vi "ModelCode_Rf.vi"(9 "BarCode":string, 11 "Data In":T1) -> (1 "ModeCode":string, 3 "Data Out":T1)   [LabVIEW 2014]
uses:
  controls/Data.ctl
panel:
  # "日期"
  # "機種名稱"
  # "機種代號"
  # "商品條碼"
  # "台"
  # "OK"
  # "NG"
  # "台"
  # "總計"
  # "台"
  # "日期"
  # "機種名稱"
  # "機種代號"
  # "商品條碼"
  # "台"
  # "OK"
  # "NG"
  # "台"
  # "總計"
  # "台"
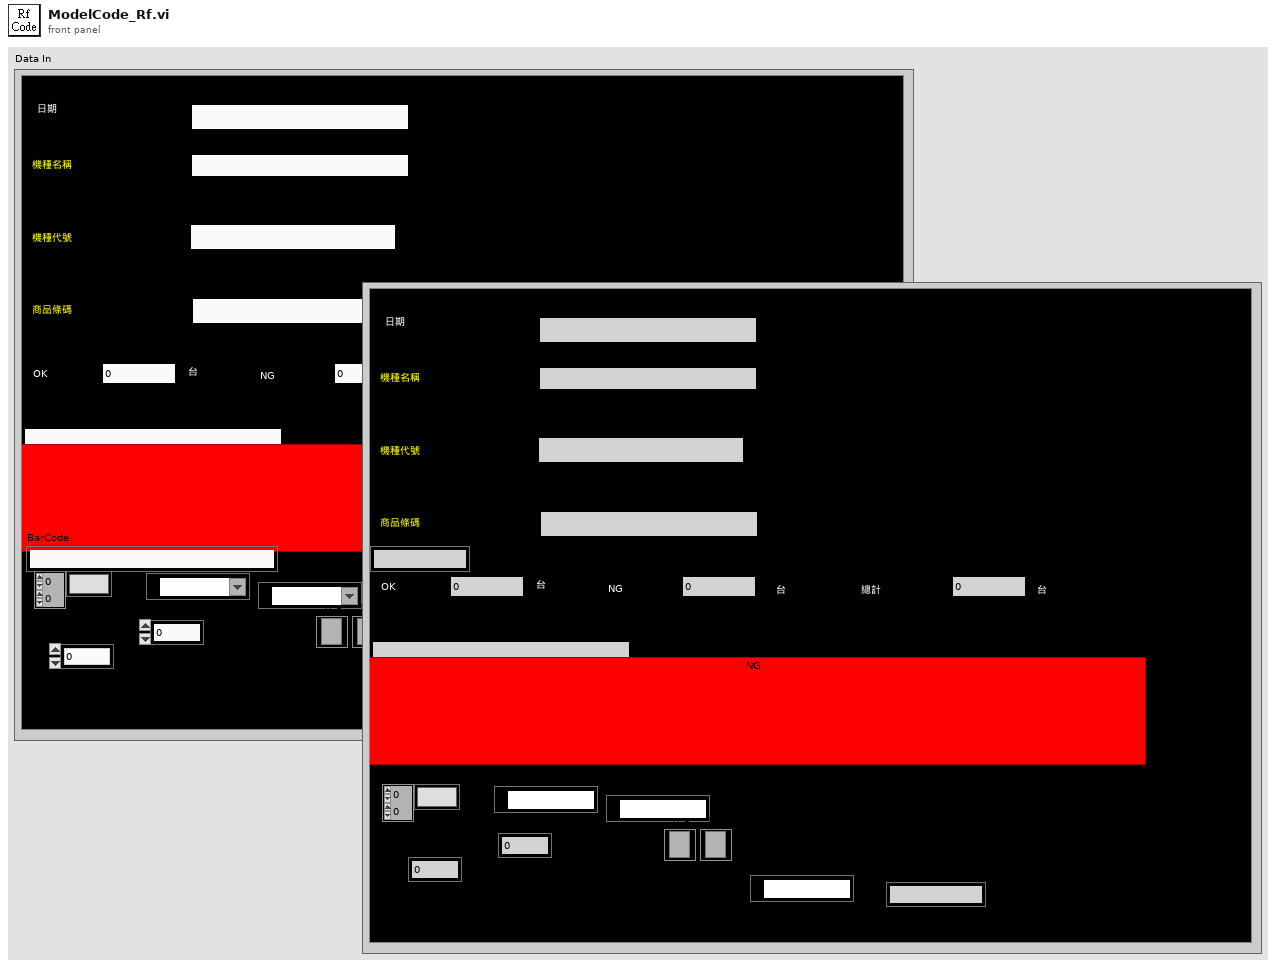
[diagram p1: front panel]
types:
  T1 = typedef "Data.ctl" = cluster{"Date":string, "BarCode1":string, "BarCode2":string, "BarCode3":string, "Message":string, "OK Count":u16, "NG Count":u16, "Total Count":u16, "ModelData":string[][], "OK&NG":bool, "COM1":refnum<visa-resource-name>, "COM2":refnum<visa-resource-name>, "IO":i32, "Time":u32, "TCP":refnum<k5>, "TCP 2":refnum<k5>, "COM3":refnum<visa-resource-name>, "CheckPars":string}
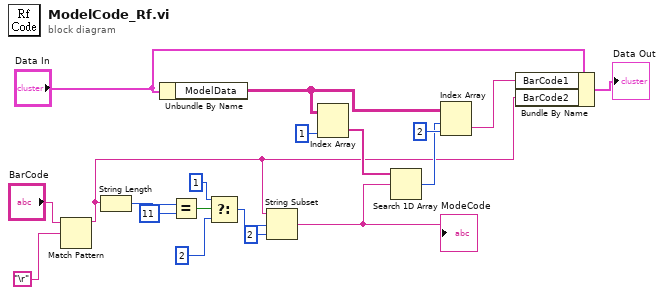
[diagram p0: block diagram]
diagram:
  n1 = Match Pattern(string="BarCode", regular expression="\r") -> (before substring=w1:string)  [unwired: 1 in, 3 out]
  n2 = String Length(string=w1) -> (length=w19:i32)
  n3 = Unbundle By Name("Data In") -> ("ModelData"=w9:string[][])
  n4 = Equal?(x=w19, y=11) -> (x = y?=w17:bool)
  n5 = Select(t=1 ("offset (0)"), s=w17, f=2) -> (s? t:f=w15:i32)
  n6 = String Subset(string=w1, offset (0)=w15, length (rest)=2 ("length (rest)")) -> (substring=w10:string)
  "ModeCode" <- w10
  n7 = Index Array(array=w9, index (col)=1 ("disabled index (col)")) -> (element=w11:string[])  [unwired: 1 in]
  n8 = Search 1D Array(1D array=w11, element=w10) -> (index of element=w7:i32)  [unwired: 1 in]
  n9 = Index Array(array=w9, index (row)=w7, index (col)=2 ("disabled index (col)")) -> (element=w4:string)
  n10 = Bundle By Name(cluster="Data In", "BarCode1"=w4, "BarCode2"=w1) -> (→"Data Out":T1)
